vi "Acknowledge ID.vi"(8 "error in (no error)":errorcluster, 10 "Packet Identifier":u16, 11 "Client in":refnum<class "Client.lvclass">) -> (0 "error out":errorcluster, 3 "Client out":refnum<class "Client.lvclass">)   [LabVIEW 2013, in "MQTT Client.lvlib" / "Client.lvclass"]
uses:
  Client.lvclass
  Client.lvclass/Client.ctl
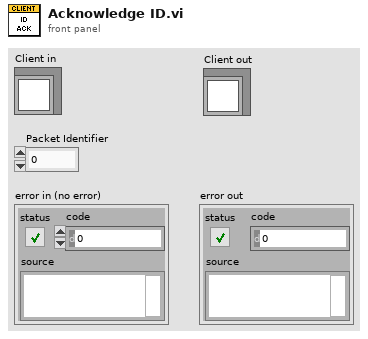
[diagram p1: front panel]
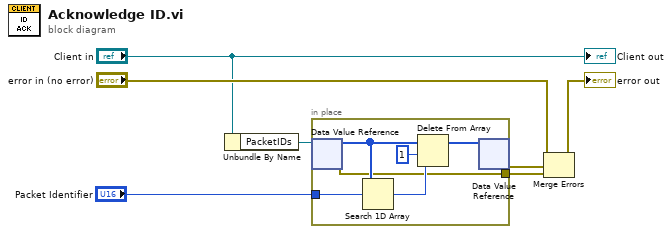
[diagram p0: block diagram]
diagram:
  n1 = Unbundle By Name("Client in") -> ("PacketIDs"=w2:refnum<data-value>)
  n2 = in-place {
    in-place-border: "Packet Identifier" -> [w13]
    in-place-border: [w8] -> w4
    n3 = in-place-dvr #1(w2) -> (w12:u16[], w8:errorcluster)
    n4 = Search 1D Array(1D array=w12, element=w13) -> (index of element=w10:i32)  [unwired: 1 in]
    n5 = Delete From Array(array=w12, length=1, index=w10) -> (array with subset deleted=w11:u16[])  [unwired: 1 out]
    n6 = in-place-dvr #1(w11) -> (w5:errorcluster)  [unwired: 1 out]
  }
  n7 = Merge Errors("error in (no error)", w5, w4) -> (→"error out":errorcluster)
  "Client out" <- "Client in"
